vi "Do.vi"(8 "Error In":errorcluster, 10 "Actor in":refnum<class "Actor.lvclass">, 11 "LNA Return Message Msg":refnum<class "LNA Return Message Msg.lvclass">) -> (0 "Error Out":errorcluster, 2 "Actor out":refnum<class "Actor.lvclass">)   [LabVIEW 2016, in "TestLNA.lvlib" / "LNA Return Message Msg.lvclass"]
doc: "(<B>Filename</B>: Actor Framework.lvlib:Message.lvclass:Do.vi)\n\nDefines what a message does when it is received by an actor. Generally, a message instructs an actor to invoke one of its methods. By default, this method does nothing. A child class must override it to define behavior. Create a child class by using the Actor Framework Message Maker dialog box."
uses:
  LNA Return Message Msg.lvclass
  <vilib>/ActorFramework/Actor/Actor.lvclass
  TestLNA.lvclass
  C:/Program Files (x86)/National Instruments/LabVIEW 2016/vi.lib/ActorFramework/Actor/Actor.lvclass
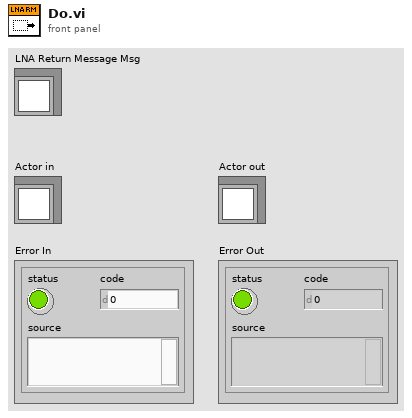
[diagram p1: front panel]
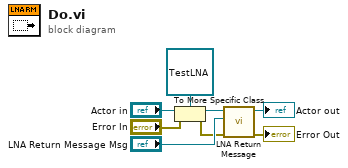
[diagram p0: block diagram]
diagram:
  n1 = To More Specific Class(target class=refnum<class "TestLNA.lvclass"> refnum ("TestLNA.lvlib:TestLNA.lvclass"), reference="Actor in", error in="Error In") -> (specific class reference=w4:refnum<class "TestLNA.lvclass">, error out=w2:errorcluster)
  n2 = call "LNA Return Message.vi"("Error In"=w2, "LNA Return Message Msg"="LNA Return Message Msg", "TestLNA in"=w4) -> ("Error Out"=→"Error Out":errorcluster, "TestLNA out"=→"Actor out":refnum<class "TestLNA.lvclass">)  [unwired: 7 in]
